vi "Intacc Immediate.vi"(6 "Position to override":dbl, 7 "Description":string, 8 "Command Info In":T1, 9 "Override position?":bool, 10 "Reverse?":bool, 11 "Intaking?":bool) -> (0 "Command Info Out":T1)   [LabVIEW 2019]
doc: "This template is useful for immediate subsystem actions that do not need deadband filtering\n\nBe sure to right-click and select New from Template and save with a new command name."
uses:
  <vilib>/Rock Robotics/WPI/Framework/Command Status Info.ctl
  <vilib>/Rock Robotics/WPI/Framework/Completion Status.ctl
  <vilib>/Rock Robotics/WPI/Framework/Completion Notifier.ctl
  Implementation/Intacc Setpoints.ctl
  Implementation/Intacc Operations.ctl
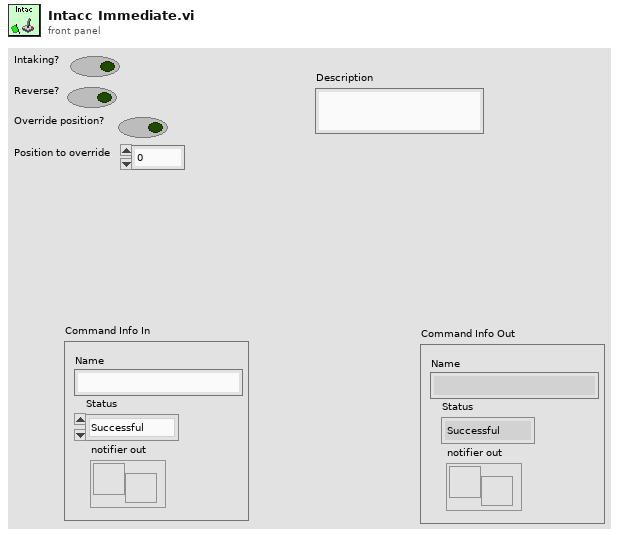
[diagram p1: front panel]
types:
  T1 = typedef "Command Status Info.ctl" = cluster{"Name":string, "Status":T2, "notifier out":T3}
  T2 = typedef "Completion Status.ctl" = enum16{"Successful", "Aborted", "Incomplete"}
  T3 = typedef "Completion Notifier.ctl" = refnum<notifier>
  T4 = typedef "Intacc Setpoints.ctl" = cluster{"Operation":T5, "Intaking?":bool, "Reverse?":bool, "Override position?":bool, "Position to override":dbl}
  T5 = typedef "Intacc Operations.ctl" = enum16{"Reserve", "Read Current", "Immediate"}
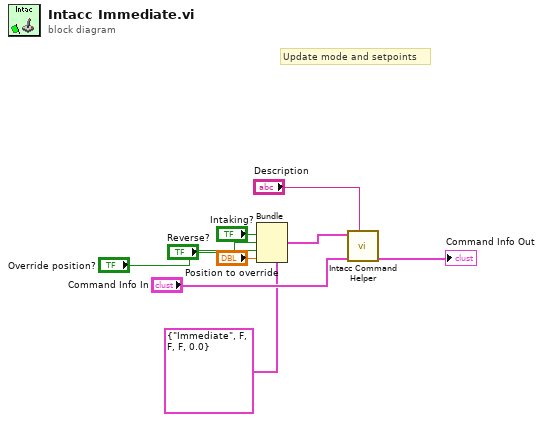
[diagram p0: block diagram]
diagram:
  # "Update mode and setpoints"
  n1 = Bundle(cluster=T4 {"Operation"=enum."Immediate", "Intaking?"=FALSE, "Reverse?"=FALSE, "Override position?"=FALSE, "Position to override"=0.0} ("SubSystem Data"), "Intaking?"="Intaking?", "Reverse?"="Reverse?", "Override position?"="Override position?", "Position to override"="Position to override") -> (w5:T4)  [unwired: 1 in]
  n2 = call "Intacc Command Helper.vi"("Description"="Description", "Command Info In"="Command Info In", "SubSystem Data"=w5) -> ("Command Info Out"=→"Command Info Out":T1)  [unwired: 6 in, 2 out]
